vi "sub_generate_data.vi"(11 "number of elements":i32) -> (2 "array items":cluster{"name":string, "address":string}[](array[cluster]), 3 "names":string[](array[string]))   [LabVIEW 2016]
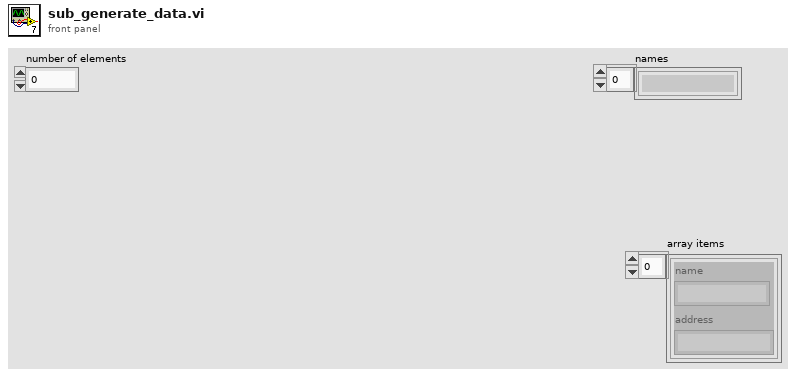
[diagram p1: front panel]
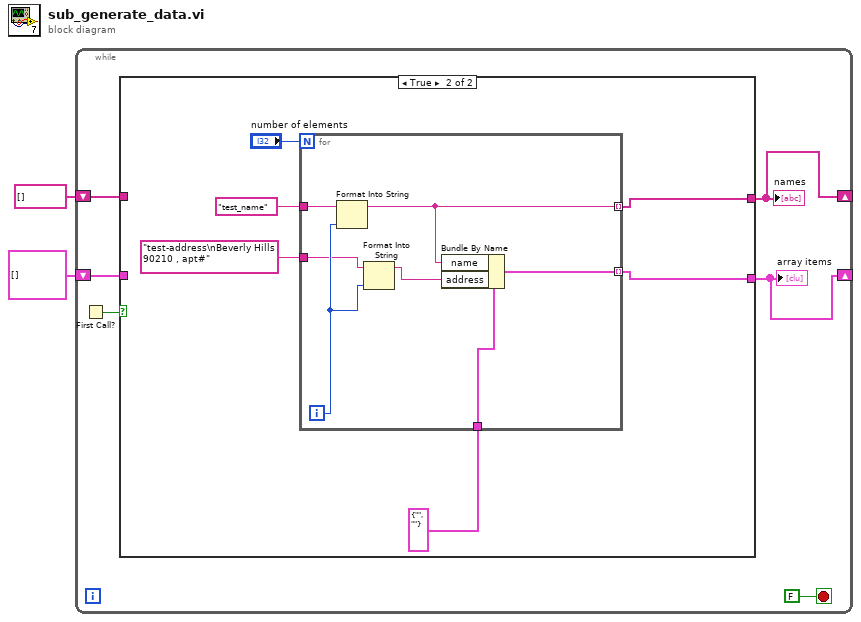
[diagram p0: block diagram]
diagram:
  n1 = while {
    shift-right: [w6] -> _
    shift-left: string[] [] -> [w4]
    shift-right: [w5] -> _
    shift-left: cluster{"name":string, "address":string}[] [] -> [w3]
    stop <- FALSE stop-if-true
    n2 = First Call?() -> (First Call?: T/F=w7:bool)
    n3 = case shown="True" w7 {
      tunnel: [w10 w12] -> w6
      tunnel: [w9 w11] -> w5
      tunnel: w4 -> [w10 _]
      tunnel: w3 -> [w9 _]
      frame False {
      }
      frame True {
        n4 = for {
          N: "number of elements" -> [_]
          tunnel: "test_name" -> [w23]
          tunnel: "test-address\nBeverly Hills 90210 , apt#" -> [w21]
          tunnel: cluster{"name":string, "address":string} {"name"="", "address"=""} ("element") -> [w20]
          tunnel: [w18] -> w11 mode=indexing
          tunnel: [w17] -> w12 mode=indexing
          i -> [w22]
          n5 = Format Into String(initial string=w23, w22) -> (resulting string=w17:string)  [unwired: 2 in, 1 out]
          n6 = Format Into String(initial string=w21, w22) -> (resulting string=w19:string)  [unwired: 2 in, 1 out]
          n7 = Bundle By Name(cluster=w20, "name"=w17, "address"=w19) -> (w18:cluster{"name":string, "address":string})
        }
      }
    }
    "names" <- w6
    "array items" <- w5
  }
